vi "PS3 Controller.vi"(8 "error in (no error)":errorcluster, 11 "device ID":refnum<k1>) -> (0 "error out":errorcluster, 1 "Arrows":i32, 2 "Buttons control":T1, 3 "Control cluster":T2 {"Roll" scale=-1.0..1.0; "Pitch" scale=-1.0..1.0; "Vertical Speed" scale=-1.0..1.0; "Yaw Speed" scale=-1.0..1.0})   [LabVIEW 2014]
uses:
  <vilib>/Utility/inputDevices.llb/joystickAcquire.vi
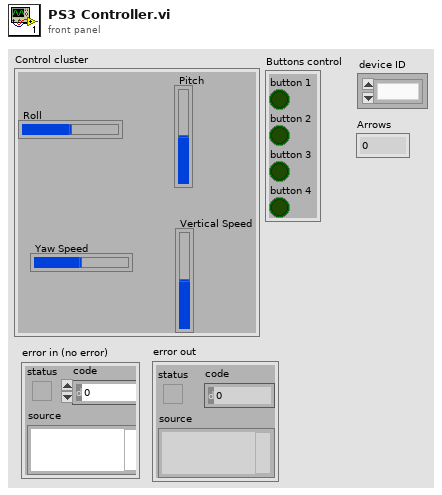
[diagram p1: front panel]
types:
  T1 = cluster{"button 1":bool, "button 2":bool, "button 3":bool, "button 4":bool}
  T2 = cluster{"Roll":dbl, "Pitch":dbl, "Vertical Speed":dbl, "Yaw Speed":dbl}
  T3 = cluster{"X axis":dbl, "Y axis":dbl, "Z axis":dbl, "X axis rotation":dbl}
  T4 = cluster{"X axis":i32, "Y axis":i32, "Z axis":i32, "X axis rotation":i32, "Y axis rotation":i32, "Z axis rotation":i32, "U axis":i32, "V axis":i32}
  T5 = cluster{"button 1":bool, "button 2":bool, "button 3":bool, "button 4":bool, "button 5":bool, "button 6":bool, "button 7":bool, "button 8":bool, "button 9":bool, "button 10":bool, "button 11":bool, "button 12":bool, "button 13":bool, "button 14":bool, "button 15":bool, "button 16":bool, "button 17":bool, "button 18":bool, "button 19":bool, "button 20":bool, "button 21":bool, "button 22":bool, "button 23":bool, "button 24":bool, "button 25":bool, "button 26":bool, "button 27":bool, "button 28":bool, "button 29":bool, "button 30":bool, "button 31":bool, "button 32":bool}
  T6 = cluster{"pov 1":i32, "pov 2":i32, "pov 3":i32, "pov 4":i32}
  T7 = cluster{"X axis":dbl, "Y axis":dbl, "Z axis":dbl, "X axis rotation":dbl, "Y axis rotation":dbl, "Z axis rotation":dbl, "U axis":dbl, "V axis":dbl}
  T8 = cluster{"X axis":sgl, "Y axis":sgl, "Z axis":sgl, "X axis rotation":sgl, "Y axis rotation":sgl, "Z axis rotation":sgl, "U axis":sgl, "V axis":sgl}
  T9 = cluster{"X axis":sgl, "Y axis":sgl, "Z axis":sgl, "X axis rotation":sgl}
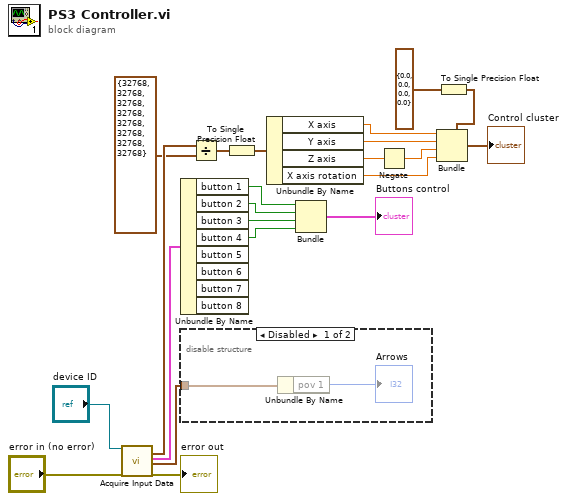
[diagram p0: block diagram]
diagram:
  n1 = call-poly <vilib>:"Acquire Input Data.vi"("device ID"="device ID", "error in (no error)"="error in (no error)") -> ("axis info"=w15:T4, "button info"=w18:T5, "direction info"=w16:T6, "error out"=→"error out":errorcluster)  [unwired: 13 in, 1 out]
  n2 = Unbundle By Name(w18) -> ("button 1"=w9:bool, "button 2"=w8:bool, "button 3"=w7:bool, "button 4"=w6:bool)  [unwired: 4 out]
  n3 = disable-structure shown="Disabled" {
    disable-tunnel: w16 -> [w23 _]
    frame Disabled {
      n4 = Unbundle By Name(w23) -> ("pov 1"=→"Arrows":i32)
    }
    frame Enabled {
    }
  }
  n5 = Divide(x=w15, y=T4 {"X axis"=32768, "Y axis"=32768, "Z axis"=32768, "X axis rotation"=32768, "Y axis rotation"=32768, "Z axis rotation"=32768, "U axis"=32768, "V axis"=32768}) -> (x/y=w4:T7)
  n6 = To Single Precision Float(number=w4) -> (single precision float=w3:T8)
  n7 = Unbundle By Name(w3) -> ("X axis"=w22:sgl, "Y axis"=w10:sgl, "Z axis"=w13:sgl, "X axis rotation"=w11:sgl)
  n8 = Bundle("button 1"=w9, "button 2"=w8, "button 3"=w7, "button 4"=w6) -> (→"Buttons control":T1)  [unwired: 1 in]
  n9 = Negate(x=w13) -> (-x=w12:sgl)
  n10 = To Single Precision Float(number=T3 {"X axis"=0.0, "Y axis"=0.0, "Z axis"=0.0, "X axis rotation"=0.0} ("cluster")) -> (single precision float=w1:T9)
  n11 = Bundle(cluster=w1, "X axis"=w22, "Y axis"=w10, "Z axis"=w12, "X axis rotation"=w11) -> (→"Control cluster":T9)
